vi "Append schedule.vi"(8 "error in (no error)":errorcluster, 10 "Monkey Schedule Message":T1, 11 "Monkey in":refnum<class "Monkey.lvclass">) -> (0 "error out":errorcluster, 3 "Monkey out":refnum<class "Monkey.lvclass">)   [LabVIEW 2020, in "Monkey.lvlib" / "Monkey.lvclass"]
uses:
  Monkey.lvclass
  Monkey.lvclass/Monkey.ctl
  Run Utilities/Run Block/Run Block.lvclass
  Run Utilities/Schedule/Schedule.lvclass
  Run Utilities/TypeDefs/DAQ Control.ctl
  Run Utilities/Run Utilities.lvlib
  Run Utilities/TypeDefs/Messages/Schedule Message.ctl
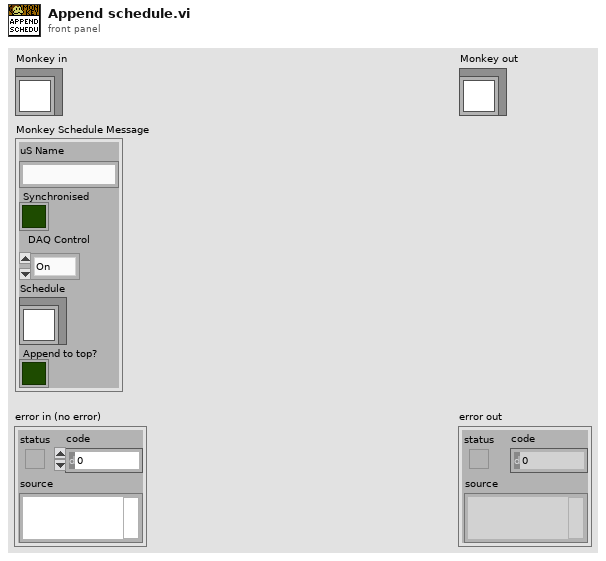
[diagram p1: front panel]
types:
  T1 = typedef "Run Utilities.lvlib/Schedule Message.ctl" = cluster{"uS Name":string, "Synchronised":bool, "DAQ Control":T2, "Schedule":refnum<class "Schedule.lvclass">, "Append to top?":bool}
  T2 = typedef "Run Utilities.lvlib/DAQ Control.ctl" = enum16{"On", "Off", "External"}
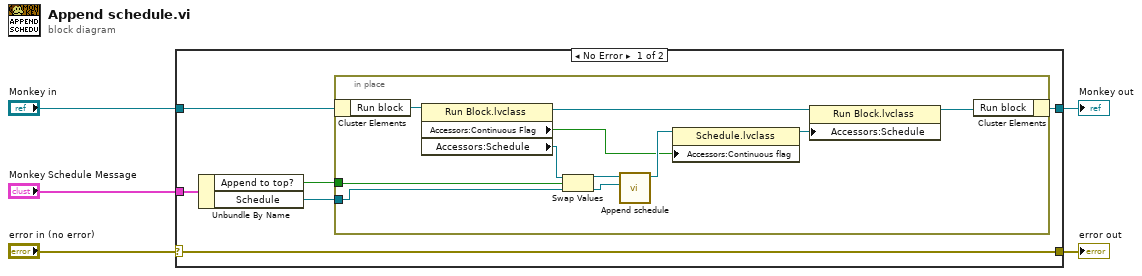
[diagram p0: block diagram]
diagram:
  n1 = case shown="No Error" "error in (no error)" {
    selector: "error in (no error)" -> [w11 w24]
    tunnel: [w11 w24] -> w4
    tunnel: [w8 w23] -> w2
    tunnel: "Monkey in" -> [w9 w23]
    tunnel: "Monkey Schedule Message" -> [w10 _]
    frame No Error {
      n2 = Unbundle By Name(w10) -> ("Append to top?"=w6:bool, "Schedule"=w7:refnum<class "Schedule.lvclass">)
      n3 = in-place {
        in-place-border: w7 -> [w18]
        in-place-border: w6 -> [w19]
        n4 = in-place-cluster #1(w9) -> ("Run block"=w22:refnum<class "Run Block.lvclass">)
        n5 = property class="Run Block.lvclass"(reference=w22) -> (reference out=w21:refnum<class "Run Block.lvclass">, "Accessors:Continuous Flag"=w12:bool, "Accessors:Schedule"=w15:refnum<class "Schedule.lvclass">)  [unwired: 1 in, 1 out]
        n6 = Swap Values(12:w15, 13:w19, 14:w18) -> (1:w17:refnum<class "Schedule.lvclass">, 3:w16:refnum<class "Schedule.lvclass">)
        n7 = call-dynamic "Append schedule.vi"("Schedule to append"=w16, "Schedule in"=w17) -> ("Schedule out"=w14:refnum<class "Schedule.lvclass">)  [unwired: 8 in, 1 out]
        n8 = property class="Schedule.lvclass"(reference=w14, "Accessors:Continuous flag"=w12) -> (reference out=w13:refnum<class "Schedule.lvclass">)  [unwired: 1 in, 1 out]
        n9 = property class="Run Block.lvclass"(reference=w21, "Accessors:Schedule"=w13) -> (reference out=w20:refnum<class "Run Block.lvclass">)  [unwired: 1 in, 1 out]
        n10 = in-place-cluster #1("Run block"=w20) -> (w8:refnum<class "Monkey.lvclass">)
      }
    }
    frame Error {
    }
  }
  "error out" <- w4
  "Monkey out" <- w2
